vi "HI-Port_XMLRelult_Save_To_File.vi"(8 "所有测试数据":string[][](array[string])=[["SN", "NA", "NA", "NA", "NA", "NA", "NA", "NA", "NA", ""], ["AC(mA)", "54", "42", "654", "354", "34", "543", "25", "45", ""], ["IR(Mohm)", "54", "42", "654", "354", "34", "543", "25", "45", ""], ["Result", "PASS", "FAIL", "PASS", "FAIL", "PASS", "FAIL", "FAIL", "FAIL", ""], ["", "", "", "", "", "", "", "", "", "NA"]], 10 "XML File Path":path caption="XML文件路径") -> (1 "数组 4":string[](array[string]), 3 "XML文件路径":path[](array[path]))   [LabVIEW 2018]
uses:
  Subvi/Global.vi
panel:
  out "value":string
  out "添加的数组":string[](array[string])
  out "fail Iteme name":string
  out "数组 3":string[](array[string])
  out "所有测试数据 2":string[](array[string])
  out "子数组 2":string[](array[string])
  out "子数组":string[](array[string])
  out "数组 2":string[](array[string])
  in  "测试数据":i32(listbox)
  out "数组":string[](array[string])
  # "1"
  # "2"
  # "3"
  # "4"
  # "5"
  # "6"
  # "7"
  # "8"
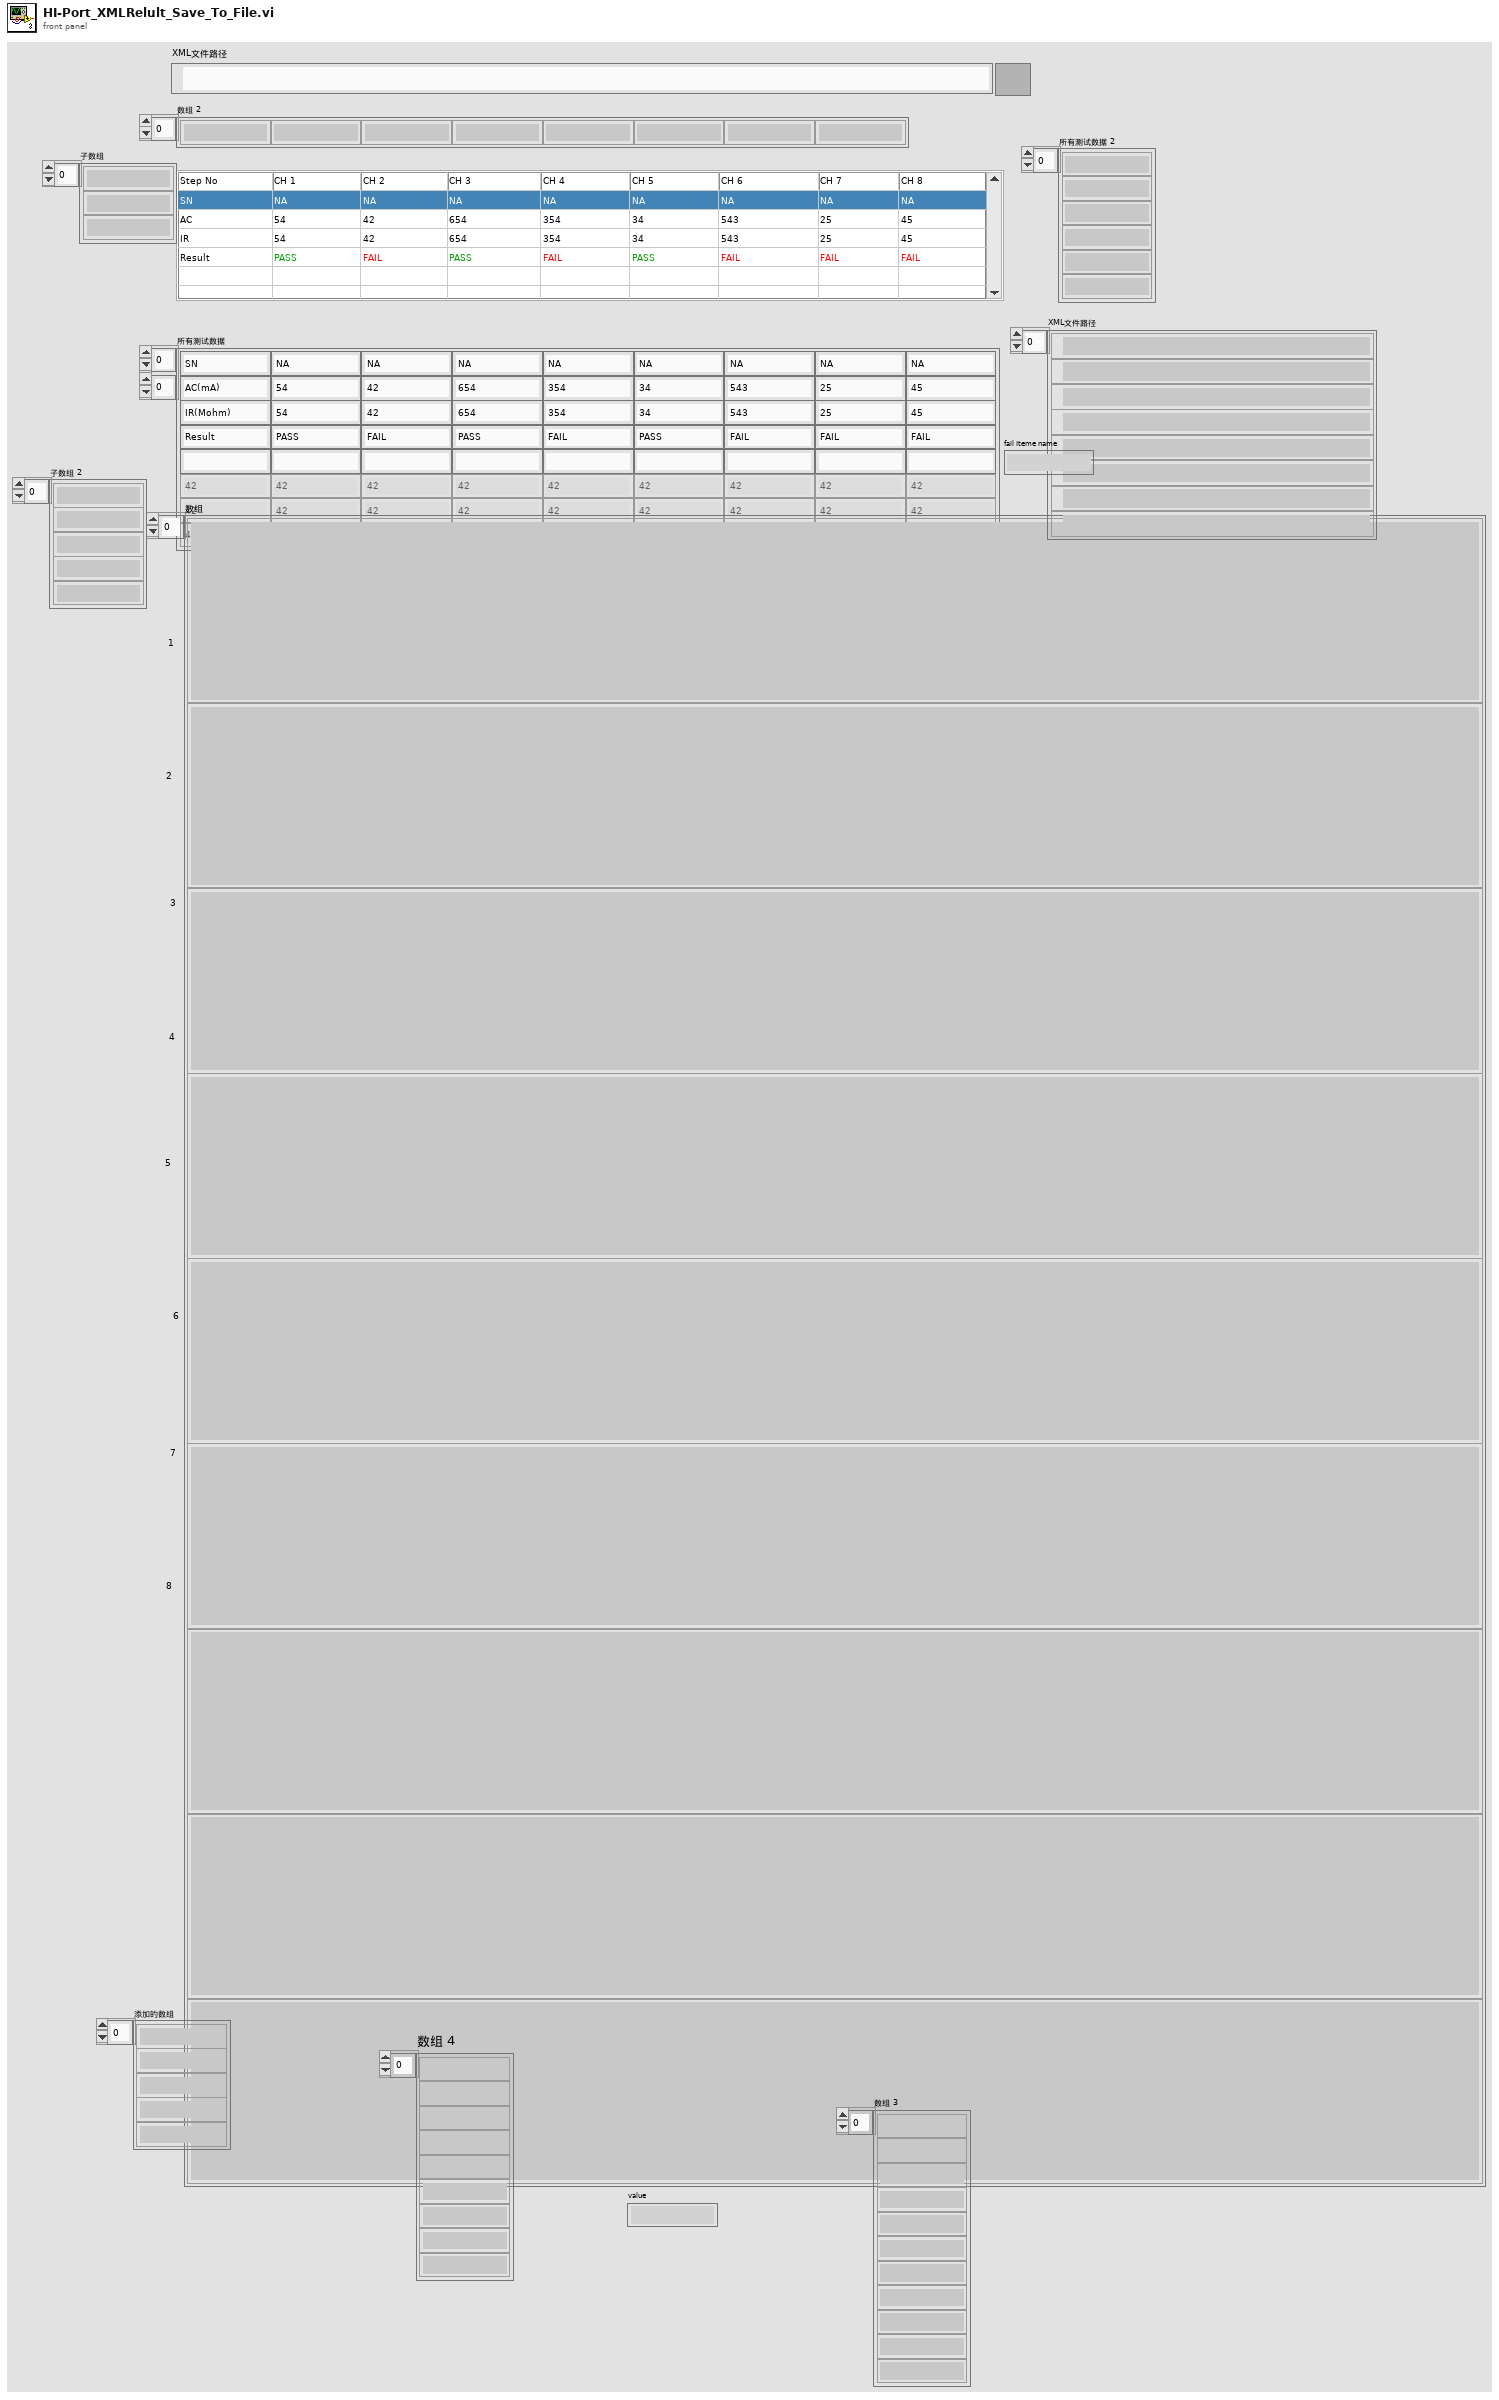
[diagram p1: front panel]
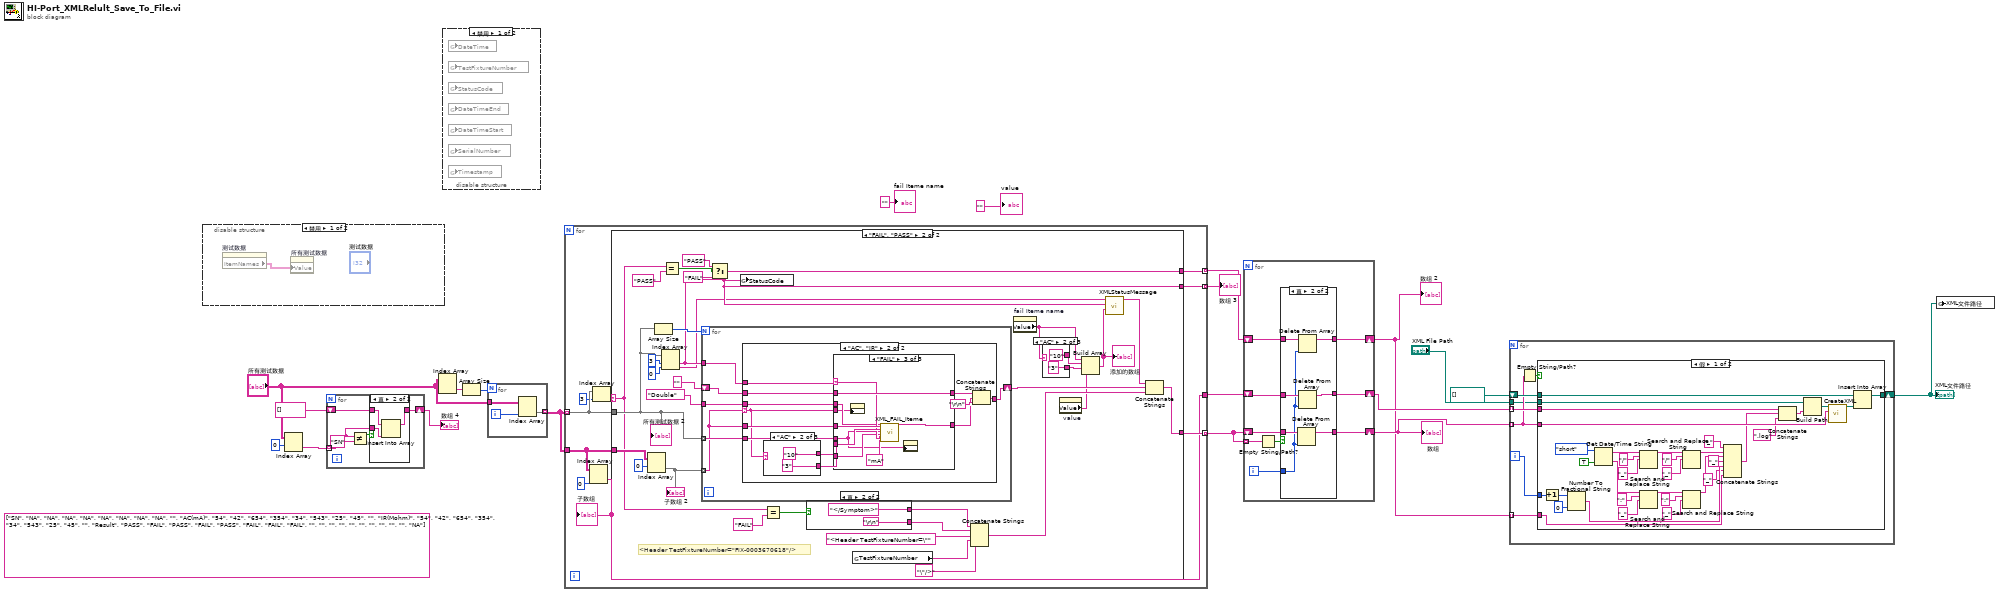
[diagram p0: block diagram]
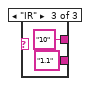
[diagram p8: hidden frame]
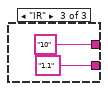
[diagram p12: hidden frame]
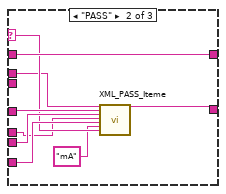
[diagram p14: hidden frame]
diagram:
  (unwired) string[][] [["SN", "NA", "NA", "NA", "NA", "NA", "NA", "NA", "NA", ""], ["AC(mA)", "54", "42", "654", "354", "34", "543", "25", "45", ""], ["IR(Mohm)", "54", "42", "654", "354", "34", "543", "25", "45", ""], ["Result", "PASS", "FAIL", "PASS", "FAIL", "PASS", "FAIL", "FAIL", "FAIL", ""], ["", "", "", "", "", "", "", "", "", "NA"]] ("所有测试数据")
  n1 = disable-structure shown="禁用" {
    frame Disabled {
      n2 = property on="测试数据" class="MCListbox (严格)"() -> ("ItemNames"=w21:string[][])  [unwired: 2 in, 2 out]
      n3 = property on="所有测试数据" class="Arr (严格)"("Value"=w21) -> ()  [unwired: 2 in, 2 out]
    }
    frame Enabled {
    }
  }
  n4 = Index Array(array="所有测试数据", index (row)=0 ("索引 (行)")) -> (element=w3:string[])  [unwired: 1 in]
  n5 = for {
    tunnel: w3 -> [w23] mode=indexing
    shift-right: [w24] -> w1
    shift-left: string[] [] -> [w25]
    n6 = Not Equal?(x=w23, y="SN") -> (x != y?=w22:bool)
    n7 = case shown="真" w22 {
      tunnel: w25 -> [_ w29]
      tunnel: [_ w28] -> w24
      tunnel: w23 -> [_ w27]
      frame False {
      }
      frame True {
        n8 = Insert Into Array(array=w29, new element=w27) -> (w28:string[])  [unwired: 1 in]
      }
    }
  }
  "数组 4" <- w1
  n9 = Index Array(array="所有测试数据") -> (element=w19:string[])  [unwired: 2 in]
  n10 = disable-structure shown="禁用" {
    frame Disabled {
      n11 = global read "Global.vi" "DateTime"() -> ()  [unwired: 1 in]
      n12 = global read "Global.vi" "TestFixtureNumber"() -> ()  [unwired: 1 in]
      n13 = global read "Global.vi" "StatusCode"() -> ()  [unwired: 1 in]
      n14 = global read "Global.vi" "DateTimeEnd"() -> ()  [unwired: 1 in]
      n15 = global read "Global.vi" "DateTimeStart"() -> ()  [unwired: 1 in]
      n16 = global read "Global.vi" "SerialNumber"() -> ()  [unwired: 1 in]
      n17 = global read "Global.vi" "Timestamp"() -> ()  [unwired: 1 in]
    }
    frame Enabled {
    }
  }
  n18 = Array Size(array=w19) -> (size(s)=w20:i32)
  n19 = for {
    N: w20 -> [_]
    tunnel: "所有测试数据" -> [w32]
    tunnel: [w31] -> w18 mode=indexing
    i -> [w30]
    n20 = Index Array(array=w32, index (col)=w30) -> (element=w31:string[])  [unwired: 1 in]
  }
  n21 = for {
    tunnel: w18 -> [w41] mode=indexing
    tunnel: w18 -> [w37]
    tunnel: [w39] -> w17 mode=indexing
    tunnel: [w36] -> w16
    tunnel: [w34] -> w11 mode=indexing
    tunnel: [w33] -> w8 mode=indexing
    n22 = Index Array(array=w37, index (col)=0 ("索引")) -> (element=w36:string[])  [unwired: 1 in]
    "子数组" <- w36
    n23 = Index Array(array=w41, index=3 ("索引")) -> (element=w38:string)
    n24 = case shown="\"FAIL\", \"PASS\"" w38 {
      selector: w38 -> [_ w47]
      tunnel: w37 -> [_ w62]
      tunnel: w41 -> [_ w56]
      tunnel: [_ w63] -> w39
      tunnel: [_ w55] -> w34
      tunnel: [_ w54] -> w33
      frame "假", Default {
      }
      frame "FAIL", "PASS" {
        # "<Header TestFixtureNumber=\"FIX-0003670618\"/>"
        n25 = Index Array(array=w62, index (row)=0 ("索引")) -> (element=w64:string[])  [unwired: 1 in]
        "子数组 2" <- w64
        n26 = Array Size(array=w56) -> (size(s)=w65:i32)
        n27 = Index Array(array=w56, index #1=3 ("索引"), index #2=0 ("索引")) -> (element #1=w54:string, element #2=w52:string)
        n28 = Equal?(x=w47, y="PASS") -> (x = y?=w58:bool)
        n29 = for {
          N: w65 -> [_]
          shift-right: [w84] -> w73
          shift-left: "" -> [w86]
          tunnel: "Double" ("组合框") -> [w85]
          tunnel: w64 -> [w82] mode=indexing
          tunnel: w56 -> [w83] mode=indexing
          tunnel: w54 -> [w81]
          n30 = case shown="\"AC\", \"IR\"" w82 {
            selector: w82 -> [_ w89]
            tunnel: w86 -> [w87 w99]
            tunnel: w85 -> [_ w98]
            tunnel: [w87 w97] -> w84
            tunnel: w81 -> [_ w96]
            tunnel: w82 -> [_ w95]
            tunnel: w83 -> [_ w94]
            frame "假", Default {
            }
            frame "AC", "IR" {
              n31 = case shown="\"AC\"" w89 {
                tunnel: [_ "3" "1.1"] -> w91
                tunnel: [_ "10" "10"] -> w90
                frame "假", Default {
                }
                frame "AC" {
                }
                frame "IR" {
                }
              }
              n32 = case shown="\"FAIL\"" w96 {
                selector: w96 -> [_ w108 w119]
                tunnel: w99 -> [w104 w112 w122]
                tunnel: [_ w113 w123] -> w92
                tunnel: w98 -> [_ w107 w117]
                tunnel: [w104 w112 w122] -> w88
                tunnel: w95 -> [_ w111 w121]
                tunnel: w94 -> [_ w106 w114]
                tunnel: w91 -> [_ w110 w118]
                tunnel: w90 -> [_ w109 w120]
                tunnel: w89 -> [_ _ w115]
                frame "假", Default {
                }
                frame "PASS" {
                  n33 = call "XML_PASS_Iteme.vi"("组合框"=w107, "Name"=w111, "UpperLimit"=w109, "Value"=w106, "LowerLimit"=w110, "MeasurementUnit"="mA", "StatusCode"=w108) -> ("连接的字符串"=w113:string)  [unwired: 20 in]
                }
                frame "FAIL" {
                  n34 = property on="fail Iteme name" class="Str"("Value"=w115) -> ()  [unwired: 2 in, 2 out]
                  n35 = call "XML_FAIL_Iteme.vi"("组合框"=w117, "Name"=w121, "UpperLimit"=w120, "Value"=w114, "LowerLimit"=w118, "MeasurementUnit"="mA", "StatusCode"=w119) -> ("连接的字符串"=w123:string)  [unwired: 20 in]
                  n36 = property on="value" class="Str"("Value"=w114) -> ()  [unwired: 2 in, 2 out]
                }
              }
              n37 = Concatenate Strings(w88, w92, "\r\n") -> (w97:string)
            }
          }
        }
        n38 = Select(t="PASS", s=w58, f="FAIL") -> (s? t:f=w55:string)
        n39 = global write "Global.vi" "StatusCode"(w54) -> ()
        n40 = Equal?(x=w47, y="FAIL") -> (x = y?=w48:bool)
        n41 = case shown="真" w48 {
          tunnel: [_ "</Symptom>"] -> w51
          tunnel: [_ "\r\n"] -> w50
          frame False {
          }
          frame True {
          }
        }
        n42 = global read "Global.vi" "TestFixtureNumber"() -> (w69:string)
        n43 = Concatenate Strings(w51, w50, "<Header TestFixtureNumber=\"", w69, "\"/>") -> (w67:string)
        n44 = property on="fail Iteme name" class="Str"() -> ("Value"=w43:string)  [unwired: 2 in, 2 out]
        n45 = case shown="\"AC\"" w43 {
          tunnel: [_ "3" "1.1"] -> w44
          tunnel: [_ "10" "10"] -> w45
          frame "假", Default {
          }
          frame "AC" {
          }
          frame "IR" {
          }
        }
        n46 = property on="value" class="Str"() -> ("Value"=w42:string)  [unwired: 2 in, 2 out]
        n47 = Build Array(w43, w45, w44, w42) -> (w46:string[])
        "添加的数组" <- w46
        n48 = call "XMLStatusMessage.vi"("数组"=w46, "StatusCode"=w54, "SerialNumber"=w52) -> ("连接的字符串"=w74:string)  [unwired: 7 in, 1 out]
        n49 = Concatenate Strings(w74, w73, w67) -> (w63:string)
        "所有测试数据 2" <- w56
      }
    }
  }
  "数组 3" <- w8
  n50 = for {
    shift-right: [w129] -> w14
    shift-left: w17 -> [w131]
    tunnel: w17 -> [w130] mode=indexing
    shift-right: [w126] -> w15
    shift-left: w16 -> [w127]
    shift-right: [w124] -> w10
    shift-left: w11 -> [w125]
    i -> [w128]
    n51 = Empty String/Path?(string/path=w130) -> (empty?=w132:bool)
    n52 = case shown="真" w132 {
      tunnel: w131 -> [w135 w142]
      tunnel: [w135 w141] -> w129
      tunnel: w128 -> [_ w138]
      tunnel: w127 -> [w134 w140]
      tunnel: [w134 w139] -> w126
      tunnel: w125 -> [w133 w137]
      tunnel: [w133 w136] -> w124
      frame False {
      }
      frame True {
        n53 = Delete From Array(array=w142, index=w138) -> (array with subset deleted=w141:string[])  [unwired: 1 in, 1 out]
        n54 = Delete From Array(array=w137, index=w138) -> (array with subset deleted=w136:string[])  [unwired: 1 in, 1 out]
        n55 = Delete From Array(array=w140, index=w138) -> (array with subset deleted=w139:string[])  [unwired: 1 in, 1 out]
      }
    }
  }
  "数组" <- w14
  "数组 2" <- w10
  n56 = for {
    tunnel: w15 -> [w150] mode=indexing
    tunnel: w14 -> [w147] mode=indexing
    shift-right: [w148] -> w9
    shift-left: path[] [] -> [w149]
    tunnel: "XML File Path" -> [w145]
    tunnel: w10 -> [w143] mode=indexing
    i -> [w144]
    n57 = Empty String/Path?(string/path=w147) -> (empty?=w146:bool)
    n58 = case shown="假" w146 {
      tunnel: w145 -> [w184 _]
      tunnel: w150 -> [w182 _]
      tunnel: w149 -> [w180 w185]
      tunnel: [w179 w185] -> w148
      tunnel: w147 -> [w177 _]
      tunnel: w144 -> [w158 _]
      tunnel: w143 -> [w151 _]
      frame False {
        n59 = Increment(x=w158) -> (x+1=w157:i32)
        n60 = Number To Fractional String(number=w157, precision (6)=i16 0 ("精度(6)")) -> (F-format string=w155:string)  [unwired: 2 in]
        n61 = Get Date/Time String(date format (0)=enum16{"short", "long", "abbreviated"}."short" ("日期格式(0)"), want seconds? (F)=TRUE ("需要秒？(F)")) -> (date string=w170:string, time string=w175:string)  [unwired: 1 in]
        n62 = Search and Replace String(input string=w170, search string="/" ("搜索字符串"), replace string="_" ("替换字符串(\"\")")) -> (result string=w172:string)  [unwired: 5 in, 3 out]
        n63 = Search and Replace String(input string=w175, search string=":" ("搜索字符串"), replace string="_" ("替换字符串(\"\")")) -> (result string=w174:string)  [unwired: 5 in, 3 out]
        n64 = Search and Replace String(input string=w172, search string="/" ("搜索字符串"), replace string="_" ("替换字符串(\"\")")) -> (result string=w171:string)  [unwired: 5 in, 3 out]
        n65 = Search and Replace String(input string=w174, search string=":" ("搜索字符串"), replace string="_" ("替换字符串(\"\")")) -> (result string=w173:string)  [unwired: 5 in, 3 out]
        n66 = Concatenate Strings("_" ("字符串"), w171, w173, "_" ("字符串"), w155, "_" ("字符串"), w151) -> (w153:string)
        n67 = Concatenate Strings(w182, w153, ".log" ("字符串")) -> (w183:string)
        n68 = Build Path(base path=w184, name or relative path=w183) -> (appended path=w181:path)
        n69 = call "CreateXML.vi"("XML Input"=w177, "XML File Path"=w181) -> ("XML File Path(duplicate)"=w178:path)  [unwired: 7 in, 2 out]
        n70 = Insert Into Array(array=w180, new element=w178) -> (w179:path[])  [unwired: 1 in]
      }
      frame True {
      }
    }
  }
  "XML文件路径" <- w9
  n71 = global write "Global.vi" "XML文件路径"(w9) -> ()
  "fail Iteme name" <- "" ("字符串")
  "value" <- "" ("字符串")
